vi "poly_h5_append_array_0d_to_1d.vi"(8 "error in":errorcluster, 10 "value":dbl, 11 "h5 1d array ref":T1 format="%.0x") -> (0 "error out":errorcluster)   [LabVIEW 2015]
uses:
  <vilib>/addons/h5labview2/base/hid_t.ctl
  <vilib>/addons/h5labview2/base/lib_path.vi
  <vilib>/addons/h5labview2/base/H5Equery.vi
  <vilib>/addons/h5labview2/dataset/H5Dwrite.llb/H5Dwrite.xnode
  <vilib>/addons/h5labview2/dataset/H5D.lvlib
  <vilib>/addons/h5labview2/space/H5S.lvlib
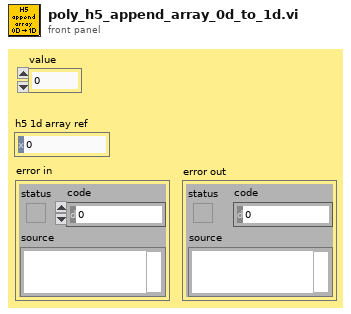
[diagram p1: front panel]
types:
  T1 = typedef "hid_t.ctl" = i32
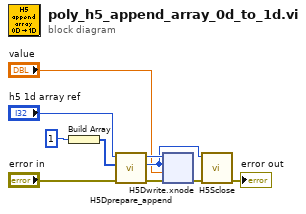
[diagram p0: block diagram]
diagram:
  n1 = Build Array(1 ("ndims")) -> (w5:i32[])
  n2 = call <vilib>:"H5Dprepare_append.vi"("error in (no error)"="error in", "append dims"=w5, "dset in"="h5 1d array ref") -> ("error out"=w8:errorcluster, "space out"=w9:T1, "dset out"=w10:T1)  [unwired: 5 in, 1 out]
  n3 = xnode "H5Dwrite.xnode"("error in (no error)"=w8, "data"="value", "file space"=w9, "ref in"=w10) -> ("error out"=w7:errorcluster)  [unwired: 3 in, 2 out]
  n4 = call <vilib>:"H5Sclose.vi"("error in (no error)"=w7, "space in"=w9) -> ("error out"=→"error out":errorcluster)  [unwired: 9 in]
